vi "SVPO Vector Average Spectrum (Complex) with IC.vi"(0 "complex spectrum [EU rms]":T7={"complex spectrum response"={"f0"=0.0, "df"=1.0, "complex spectrum"=[]}, "spectrum info"={"channel name"="", "description"="", "x-axis units"=0, "spectral info"={"spectrum type"=enum."Power [Magnitude^2]", "linear/dB"=enum."linear", "window"=0, "window size"=0, "FFT size"=0}, "engineering units"=0, "custom label"="", "dB reference [EU]"=0.0, "peak units"=enum."rms", "weighting filter"=0, "spectral density?"=FALSE, "unit label"="", "spectrum skewed?"=FALSE, "complimentary spectrum units"=enum."none"}} {"spectrum info"."x-axis units" items=["Time (s)"=0, "Frequency-CB (Hz)"=1, "Frequency-CPB (Hz)"=1248, "Frequency-Arbitrary (Hz)"=2357, "Quefrency (s)"=2, "Revolutions (rev)"=3, "Order"=4, "Speed (RPM)"=11, "Speed (rad/s)"=21, "Index"=65535]; "spectrum info"."weighting filter" items=["Linear", "A-weighting", "B-weighting", "C-weighting", "ITU-R 468-4", "Dolby", "CCITT", "C-message", "Wb", "Wc", "Wd", "We", "Wf", "Wh", "Wj", "Wk", "Wm", "AES17 20 kHz lowpass", "AES17 40 kHz lowpass", "AES17 20 kHz highpass", "AES17 40 kHz highpass"]; "spectrum info"."dB reference [EU]" format="%.2f"; "spectrum info"."engineering units" items=["custom..."=0, "V"=1, "A"=21, "C"=30, "pC"=31, "s"=32, "-"=29, "Pa"=2, "N"=20, "g"=3, "m/s^2"=4, "m/s"=5, "m"=6, "mm/s"=12, "mm"=13, "micron/s"=14, "micron"=15, "in/s^2"=7, "in/s"=8, "in"=9, "mil/s"=10, "mil"=11, "rad/s^2"=16, "rad/s"=17, "rad"=18, "deg/s^2"=26, "deg/s"=27, "deg"=28, "RPM"=22, "cycle/s^2"=23, "Hz"=24, "cycle"=25, "strain"=19]; "spectrum info"."spectral info"."window" items=["None "=0, "Hanning"=1, "Hamming"=2, "Blackman-Harris"=3, "Exact Blackman"=4, "Blackman"=5, "Flat Top"=6, "4 Term B-Harris "=7, "7 Term B-Harris"=8, "Low Sidelobe"=9, "Force - Exponential"=10, "Gaussian"=62]; "complex spectrum response"."complex spectrum" format="%.2f"; "complex spectrum response"."df" format="%.2f"; "complex spectrum response"."f0" format="%.2f"}, 3 "averaging weighting mode":enum16{"Linear", "Exponential"}(ring), 5 "average complex spectrum in":T7={"complex spectrum response"={"f0"=0.0, "df"=1.0, "complex spectrum"=[]}, "spectrum info"={"channel name"="", "description"="", "x-axis units"=0, "spectral info"={"spectrum type"=enum."Power [Magnitude^2]", "linear/dB"=enum."linear", "window"=0, "window size"=0, "FFT size"=0}, "engineering units"=0, "custom label"="", "dB reference [EU]"=0.0, "peak units"=enum."rms", "weighting filter"=0, "spectral density?"=FALSE, "unit label"="", "spectrum skewed?"=FALSE, "complimentary spectrum units"=enum."none"}} {"spectrum info"."x-axis units" items=["Time (s)"=0, "Frequency-CB (Hz)"=1, "Frequency-CPB (Hz)"=1248, "Frequency-Arbitrary (Hz)"=2357, "Quefrency (s)"=2, "Revolutions (rev)"=3, "Order"=4, "Speed (RPM)"=11, "Speed (rad/s)"=21, "Index"=65535]; "spectrum info"."weighting filter" items=["Linear", "A-weighting", "B-weighting", "C-weighting", "ITU-R 468-4", "Dolby", "CCITT", "C-message", "Wb", "Wc", "Wd", "We", "Wf", "Wh", "Wj", "Wk", "Wm", "AES17 20 kHz lowpass", "AES17 40 kHz lowpass", "AES17 20 kHz highpass", "AES17 40 kHz highpass"]; "spectrum info"."dB reference [EU]" format="%.2f"; "spectrum info"."engineering units" items=["custom..."=0, "V"=1, "A"=21, "C"=30, "pC"=31, "s"=32, "-"=29, "Pa"=2, "N"=20, "g"=3, "m/s^2"=4, "m/s"=5, "m"=6, "mm/s"=12, "mm"=13, "micron/s"=14, "micron"=15, "in/s^2"=7, "in/s"=8, "in"=9, "mil/s"=10, "mil"=11, "rad/s^2"=16, "rad/s"=17, "rad"=18, "deg/s^2"=26, "deg/s"=27, "deg"=28, "RPM"=22, "cycle/s^2"=23, "Hz"=24, "cycle"=25, "strain"=19]; "spectrum info"."spectral info"."window" items=["None "=0, "Hanning"=1, "Hamming"=2, "Blackman-Harris"=3, "Exact Blackman"=4, "Blackman"=5, "Flat Top"=6, "4 Term B-Harris "=7, "7 Term B-Harris"=8, "Low Sidelobe"=9, "Force - Exponential"=10, "Gaussian"=62]; "complex spectrum response"."complex spectrum" format="%.2f"; "complex spectrum response"."df" format="%.2f"; "complex spectrum response"."f0" format="%.2f"}, 6 "exponential weight (10 %)":dbl=10.0 min=0.0 max=100.0 step=5.0, 7 "averages completed in":dbl, 9 "restart averaging (F)":bool) -> (13 "averages completed out":dbl, 19 "average complex spectrum out":T7={"complex spectrum response"={"f0"=0.0, "df"=1.0, "complex spectrum"=[]}, "spectrum info"={"channel name"="", "description"="", "x-axis units"=0, "spectral info"={"spectrum type"=enum."Power [Magnitude^2]", "linear/dB"=enum."linear", "window"=0, "window size"=0, "FFT size"=0}, "engineering units"=0, "custom label"="", "dB reference [EU]"=0.0, "peak units"=enum."rms", "weighting filter"=0, "spectral density?"=FALSE, "unit label"="", "spectrum skewed?"=FALSE, "complimentary spectrum units"=enum."none"}} {"spectrum info"."x-axis units" items=["Time (s)"=0, "Frequency-CB (Hz)"=1, "Frequency-CPB (Hz)"=1248, "Frequency-Arbitrary (Hz)"=2357, "Quefrency (s)"=2, "Revolutions (rev)"=3, "Order"=4, "Speed (RPM)"=11, "Speed (rad/s)"=21, "Index"=65535]; "spectrum info"."weighting filter" items=["Linear", "A-weighting", "B-weighting", "C-weighting", "ITU-R 468-4", "Dolby", "CCITT", "C-message", "Wb", "Wc", "Wd", "We", "Wf", "Wh", "Wj", "Wk", "Wm", "AES17 20 kHz lowpass", "AES17 40 kHz lowpass", "AES17 20 kHz highpass", "AES17 40 kHz highpass"]; "spectrum info"."dB reference [EU]" format="%.2f"; "spectrum info"."engineering units" items=["custom..."=0, "V"=1, "A"=21, "C"=30, "pC"=31, "s"=32, "-"=29, "Pa"=2, "N"=20, "g"=3, "m/s^2"=4, "m/s"=5, "m"=6, "mm/s"=12, "mm"=13, "micron/s"=14, "micron"=15, "in/s^2"=7, "in/s"=8, "in"=9, "mil/s"=10, "mil"=11, "rad/s^2"=16, "rad/s"=17, "rad"=18, "deg/s^2"=26, "deg/s"=27, "deg"=28, "RPM"=22, "cycle/s^2"=23, "Hz"=24, "cycle"=25, "strain"=19]; "spectrum info"."spectral info"."window" items=["None "=0, "Hanning"=1, "Hamming"=2, "Blackman-Harris"=3, "Exact Blackman"=4, "Blackman"=5, "Flat Top"=6, "4 Term B-Harris "=7, "7 Term B-Harris"=8, "Low Sidelobe"=9, "Force - Exponential"=10, "Gaussian"=62]; "complex spectrum response"."complex spectrum" format="%.2f"; "complex spectrum response"."df" format="%.2f"; "complex spectrum response"."f0" format="%.2f"})   [LabVIEW 2017]
doc: "Converts a frequency power spectrum to an order power spectrum. Use this VI to convert power spectrum results from constant-speed applications."
uses:
  <vilib>/addons/_NISVFA/_Shared subVIs/Controls/svc_Spectrum Info.ctl
  <vilib>/addons/_NISVFA/_Shared subVIs/Controls/svc_X-Axis Units.ctl
  <vilib>/addons/_NISVFA/_Shared subVIs/Controls/svc_Spectrum Type.ctl
  <vilib>/addons/_NISVFA/_Shared subVIs/Controls/svc_Engineering Units Text Ring.ctl
  <vilib>/addons/_NISVFA/_Shared subVIs/Controls/svc_Weighting Filter Text Ring.ctl
  <vilib>/addons/_NISVFA/_Shared subVIs/Controls/svc_Complimentary Spectrum Units.ctl
  <vilib>/addons/_NISVFA/_Shared subVIs/Common/sv_Get NI Property Name String.vi
  <vilib>/addons/_NISVFA/_Shared subVIs/Spectrum Info/sfva_Set SV Info in Spectrum Info Description.vi
  <vilib>/addons/_NISVFA/_Shared subVIs/Spectrum Info/sfva_Get SV Info from Spectrum Info Description.vi
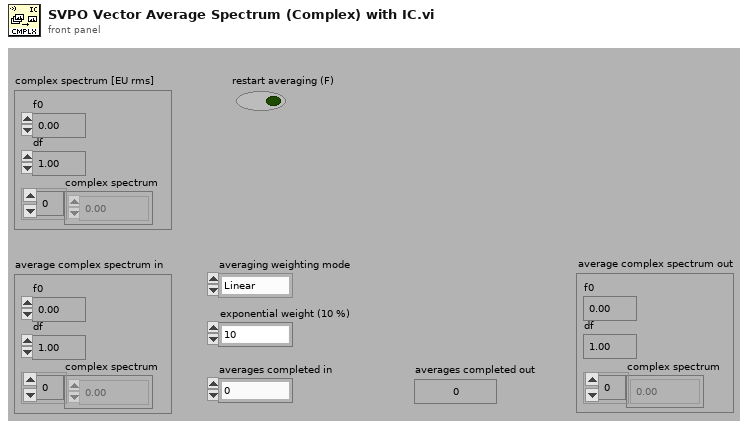
[diagram p1: front panel]
types:
  T1 = typedef "svc_Spectrum Info.ctl" = cluster{"channel name":string, "description":string, "x-axis units":T2, "spectral info":cluster{"spectrum type":T3, "linear/dB":enum16{"linear", "dB"}, "window":u16, "window size":i32, "FFT size":i32}, "engineering units":T4, "custom label":string, "dB reference [EU]":dbl, "peak units":enum16{"rms", "peak", "peak-peak"}, "weighting filter":T5, "spectral density?":bool, "unit label":string, "spectrum skewed?":bool, "complimentary spectrum units":T6}
  T2 = typedef "svc_X-Axis Units.ctl" = u16
  T3 = typedef "svc_Spectrum Type.ctl" = enum16{"FFT Spectrum [complex]", "Amplitude [Magnitude]", "Power [Magnitude^2]", "Cross Spectrum [complex]", "Frequency Response [Complex]"}
  T4 = typedef "svc_Engineering Units Text Ring.ctl" = u16
  T5 = typedef "svc_Weighting Filter Text Ring.ctl" = u16
  T6 = typedef "svc_Complimentary Spectrum Units.ctl" = enum16{"none", "radians", "degrees", "cycles", "imaginary"}
  T7 = cluster{"complex spectrum response":cluster{"f0":dbl, "df":dbl, "complex spectrum":cdb[]}, "spectrum info":T1}
  T8 = enum16{"No averaging", "Vector averaging", "RMS averaging", "Peak hold"}
  T9 = enum16{"No averaging", "Vector averaging", "RMS averaging", "Peak hold"}[]
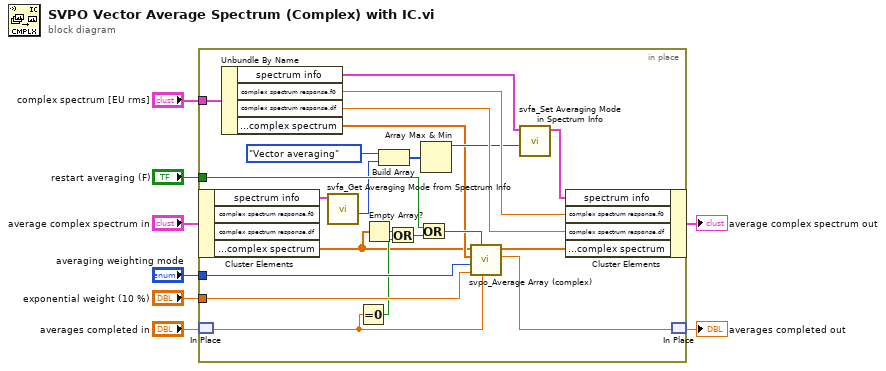
[diagram p0: block diagram]
diagram:
  n1 = in-place {
    in-place-border: "complex spectrum [EU rms]" -> [w28]
    in-place-border: "restart averaging (F)" -> [w23]
    in-place-border: "averaging weighting mode" -> [w27]
    in-place-border: "exponential weight (10 %)" -> [w26]
    n2 = in-place-cluster #1("average complex spectrum in") -> ("spectrum info"=w15:T1, "complex spectrum response.complex spectrum"=w9:cdb[])  [unwired: 2 out]
    n3 = in-place-match #2("averages completed in") -> (w22:dbl)
    n4 = Unbundle By Name(w28) -> ("spectrum info"=w17:T1, "complex spectrum response.f0"=w25:dbl, "complex spectrum response.df"=w24:dbl, "complex spectrum response.complex spectrum"=w10:cdb[])
    n5 = call <vilib>:"svfa_Get Averaging Mode from Spectrum Info.vi"("spectrum info"=w15) -> ("averaging mode"=w14:T8)  [unwired: 8 in, 2 out]
    n6 = Equal To 0?(x=w22) -> (x = 0?=w21:bool)
    n7 = Empty Array?(array=w9) -> (empty?=w20:bool)
    n8 = Build Array(T8."Vector averaging" ("averaging mode"), w14) -> (w12:T9)
    n9 = Or(x=w20, y=w21) -> (x .or. y?=w19:bool)
    n10 = Or(x=w23, y=w19) -> (x .or. y?=w18:bool)
    n11 = Array Max & Min(array=w12) -> (max value=w11:T8)  [unwired: 3 out]
    n12 = call <vilib>:"svpo_Average Array (complex).vi"("averages completed in"=w22, "restart averaging"=w18, "exponential weight (10 %)"=w26, "weighting mode"=w27, "array"=w10, "previous average array"=w9) -> ("averages completed out"=w29:dbl, "average array"=w30:cdb[])  [unwired: 4 in]
    n13 = call <vilib>:"svfa_Set Averaging Mode in Spectrum Info.vi"("averaging mode"=w11, "spectrum info in"=w17) -> ("spectrum info out"=w16:T1)  [unwired: 8 in, 1 out]
    n14 = in-place-cluster #1("spectrum info"=w16, "complex spectrum response.f0"=w25, "complex spectrum response.df"=w24, "complex spectrum response.complex spectrum"=w30) -> (→"average complex spectrum out":T7)
    n15 = in-place-match #2(w29) -> (→"averages completed out":dbl)
  }
